vi "Constants info to String Arrays.vi"(11 "Constants Info":T1[](array[typedef])) -> (2 "Constant Info Results Str":string[][](array[string]), 3 "VI Names":string[](array[string]))   [LabVIEW 2020, in "ConstantErrorsMaker.lvlib"]
uses:
  ConstantErrorsMaker.lvlib
  Constant Info--cluster.ctl
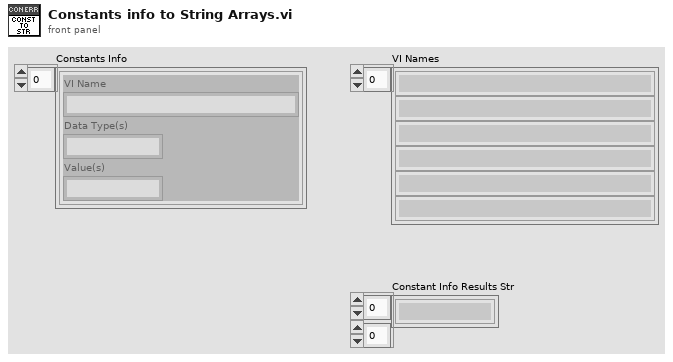
[diagram p1: front panel]
types:
  T1 = typedef "ConstantErrorsMaker.lvlib/Constant Info--cluster.ctl" = cluster{"VI Name":string, "Data Type(s)":string, "Value(s)":string}
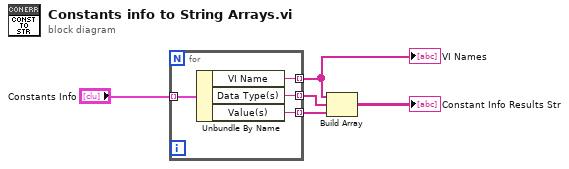
[diagram p0: block diagram]
diagram:
  n1 = for {
    tunnel: "Constants Info" -> [w9] mode=indexing
    tunnel: [w8] -> w4 mode=indexing
    tunnel: [w7] -> w3 mode=indexing
    tunnel: [w6] -> w2 mode=indexing
    n2 = Unbundle By Name(w9) -> ("VI Name"=w8:string, "Data Type(s)"=w7:string, "Value(s)"=w6:string)
  }
  "VI Names" <- w4
  n3 = Build Array(w4, w3, w2) -> (→"Constant Info Results Str":string[][])
